vi "PCO_UserInterfaceInfo.vi"() -> (0 "PCO_UserInterfaceInfo":T1, 1 "PCO_UserInterfaceInfo_Raw":T2, 2 "Length":u16, 3 "Raw_Length":u16)   [LabVIEW 2019, in "SDK.lvlib" / "Structures.lvlib"]
doc: "Use this template to build a VI to use as a subVI."
uses:
  Structures.lvlib
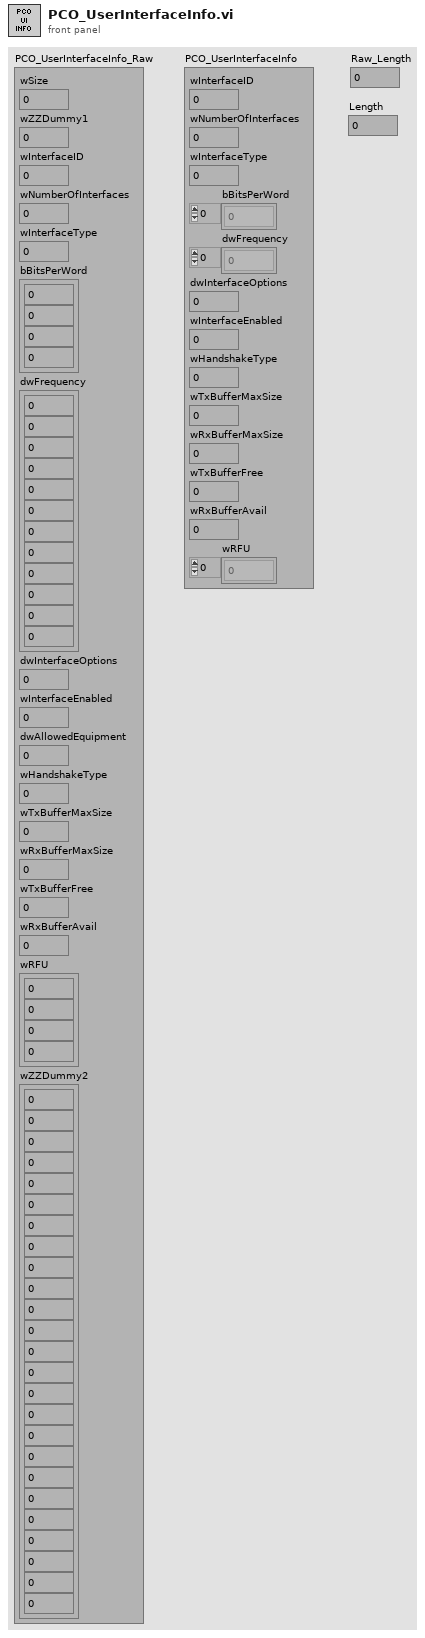
[diagram p1: front panel]
types:
  T1 = cluster{"wInterfaceID":u16, "wNumberOfInterfaces":u16, "wInterfaceType":u16, "bBitsPerWord":u8[], "dwFrequency":u32[], "dwInterfaceOptions":u32, "wInterfaceEnabled":u16, "wHandshakeType":u16, "wTxBufferMaxSize":u16, "wRxBufferMaxSize":u16, "wTxBufferFree":u16, "wRxBufferAvail":u16, "wRFU":u16[]}
  T2 = cluster{"wSize":u16, "wZZDummy1":u16, "wInterfaceID":u16, "wNumberOfInterfaces":u16, "wInterfaceType":u16, "bBitsPerWord":cluster{u8, u8, u8, u8}, "dwFrequency":cluster{u32, u32, u32, u32, u32, u32, u32, u32, u32, u32, u32, u32}, "dwInterfaceOptions":u32, "wInterfaceEnabled":u16, "dwAllowedEquipment":u32, "wHandshakeType":u16, "wTxBufferMaxSize":u16, "wRxBufferMaxSize":u16, "wTxBufferFree":u16, "wRxBufferAvail":u16, "wRFU":cluster{u16, u16, u16, u16}, "wZZDummy2":cluster{u16, u16, u16, u16, u16, u16, u16, u16, u16, u16, u16, u16, u16, u16, u16, u16, u16, u16, u16, u16, u16, u16, u16, u16, u16}}
  T3 = cluster{u32, u32, u32, u32, u32, u32, u32, u32, u32, u32, u32, u32}
  T4 = cluster{u16, u16, u16, u16, u16, u16, u16, u16, u16, u16, u16, u16, u16, u16, u16, u16, u16, u16, u16, u16, u16, u16, u16, u16, u16}
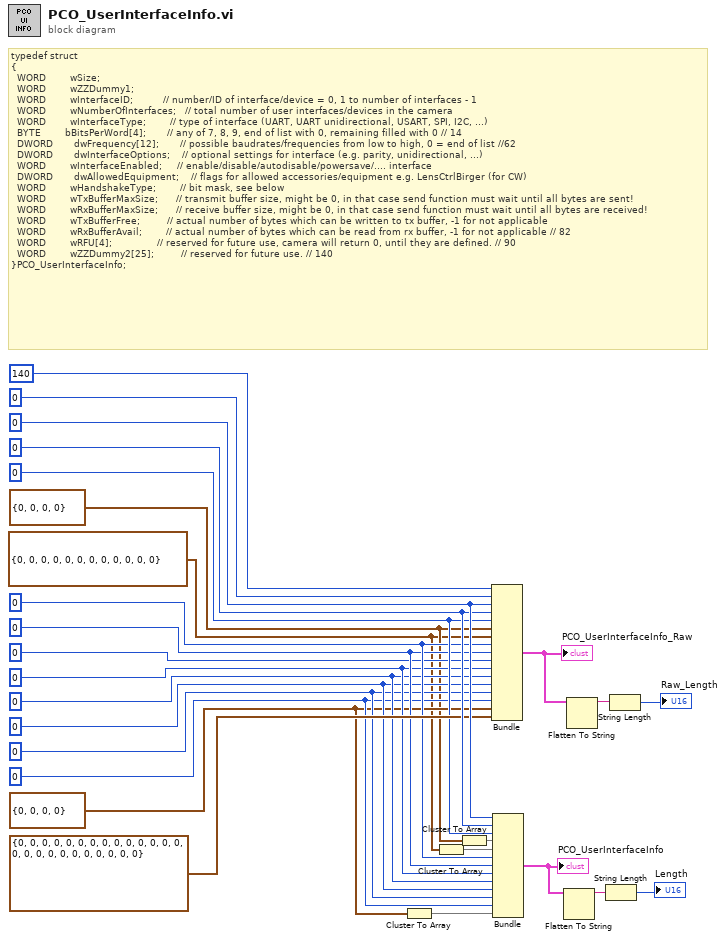
[diagram p0: block diagram]
diagram:
  w2 = T3 {0, 0, 0, 0, 0, 0, 0, 0, 0, 0, 0, 0} ("dwFrequency")
  w4 = cluster{u8, u8, u8, u8} {0, 0, 0, 0} ("bBitsPerWord")
  w6 = cluster{u16, u16, u16, u16} {0, 0, 0, 0} ("wRFU")
  w8 = u16 0 ("wRxBufferAvail")
  w9 = u16 0 ("wTxBufferFree")
  w10 = u16 0 ("wRxBufferMaxSize")
  w11 = u16 0 ("wTxBufferMaxSize")
  w12 = u16 0 ("wHandshakeType")
  w14 = u16 0 ("wInterfaceEnabled")
  w15 = u32 0 ("dwInterfaceOptions")
  w16 = u16 0 ("wInterfaceType")
  w19 = u16 0 ("wNumberOfInterfaces")
  w20 = u16 0 ("wInterfaceID")
  # "typedef struct\n{\n  WORD        wSize;\n  WORD        wZZDummy1;\n  WORD        wInterfaceID;          // number/ID of interface/device = 0, 1 to number of interfaces - 1\n  WORD        wNumberOfInterfaces;   // total number of user interfaces/devices in the camera \n  WORD        wInterfaceType;        // type of interface (UART, UART unidirectional, USART, SPI, I2C, ...)\n  BYTE        bBitsPerWord[4];       // any of 7, 8, 9, end of list with 0, remaining filled with 0 // 14\n  DWORD       dwFrequency[12];       // possible baudrates/frequencies from low to high, 0 = end of list //62\n  DWORD       dwInterfaceOptions;    // optional settings for interface (e.g. parity, unidirectional, ...)\n  WORD        wInterfaceEnabled;     // enable/disable/autodisable/powersave/.... interface \n  DWORD       dwAllowedEquipment;    // flags for allowed accessories/equipment e.g. LensCtrlBirger (for CW) \n  WORD        wHandshakeType;        // bit mask, see below\n  WORD        wTxBufferMaxSize;      // transmit buffer size, might be 0, in that case send function must wait until all bytes are sent!\n  WORD        wRxBufferMaxSize;      // receive buffer size, might be 0, in that case send function must wait until all bytes are received! \n  WORD        wTxBufferFree;         // actual number of bytes which can be written to tx buffer, -1 for not applicable\n  WORD        wRxBufferAvail;        // actual number of bytes which can be read from rx buffer, -1 for not applicable // 82\n  WORD        wRFU[4];               // reserved for future use, camera will return 0, until they are defined. // 90\n  WORD        wZZDummy2[25];         // reserved for future use. // 140\n}PCO_UserInterfaceInfo;"
  n1 = Cluster To Array(cluster=w6) -> (array=w5:u16[])
  n2 = Cluster To Array(cluster=w2) -> (array=w1:u32[])
  n3 = Cluster To Array(cluster=w4) -> (array=w3:u8[])
  n4 = Bundle("wSize"=u16 140, "wZZDummy1"=u16 0, "wInterfaceID"=w20, "wNumberOfInterfaces"=w19, "wInterfaceType"=w16, "bBitsPerWord"=w4, "dwFrequency"=w2, "dwInterfaceOptions"=w15, "wInterfaceEnabled"=w14, "dwAllowedEquipment"=u32 0, "wHandshakeType"=w12, "wTxBufferMaxSize"=w11, "wRxBufferMaxSize"=w10, "wTxBufferFree"=w9, "wRxBufferAvail"=w8, "wRFU"=w6, "wZZDummy2"=T4 {0, 0, 0, 0, 0, 0, 0, 0, 0, 0, 0, 0, 0, 0, 0, 0, 0, 0, 0, 0, 0, 0, 0, 0, 0}) -> (w21:T2)  [unwired: 1 in]
  "PCO_UserInterfaceInfo_Raw" <- w21
  n5 = Bundle("wInterfaceID"=w20, "wNumberOfInterfaces"=w19, "wInterfaceType"=w16, "bBitsPerWord"=w3, "dwFrequency"=w1, "dwInterfaceOptions"=w15, "wInterfaceEnabled"=w14, "wHandshakeType"=w12, "wTxBufferMaxSize"=w11, "wRxBufferMaxSize"=w10, "wTxBufferFree"=w9, "wRxBufferAvail"=w8, "wRFU"=w5) -> (w7:T1)  [unwired: 1 in]
  "PCO_UserInterfaceInfo" <- w7
  n6 = Flatten To String(anything=w7) -> (data string=w26:string)  [unwired: 3 in, 2 out]
  n7 = Flatten To String(anything=w21) -> (data string=w25:string)  [unwired: 3 in, 2 out]
  n8 = String Length(string=w26) -> (length=→"Length":i32)
  n9 = String Length(string=w25) -> (length=→"Raw_Length":i32)
